vi "Position_ESP300.vi"() -> ()   [LabVIEW 2012, in "ESP300.lvlib"]
uses:
  ESP300.lvlib
panel:
  in  "tickcount_pos":u32
  out "Moving":bool
  in  "Position_ESP":dbl[](array[numeric]) caption="Position" format="%.4f"
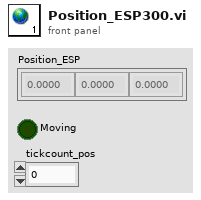
[diagram p1: front panel]
diagram:
